vi "Test - SubVI Placeholder.vi"(10 "Array":dbl[](array[numeric])) -> (2 "Numeric":dbl)   [LabVIEW 2023]
doc: "This VI is used by the Creating New VI From Template.vi example."
panel:
  # "This VI serves as a placeholder object in the template for the Creating New VI From Template.vi example."
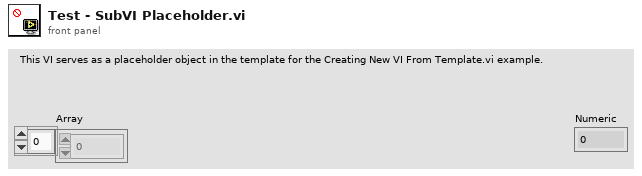
[diagram p1: front panel]
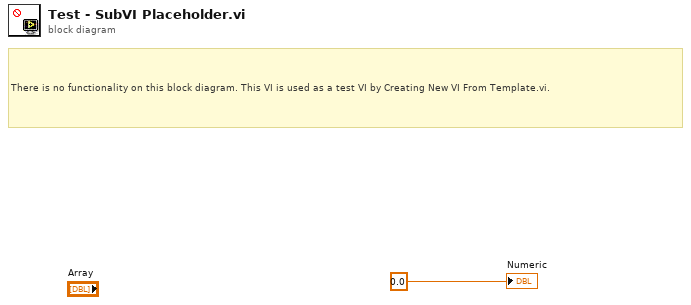
[diagram p0: block diagram]
diagram:
  # "There is no functionality on this block diagram. This VI is used as a test VI by Creating New VI From Template.vi."
  "Numeric" <- 0.0 ("Numeric")
